vi "Equal Type Comparison.vi"(8 "error in (no error)":errorcluster, 9 "Y":variant, 10 "X":variant) -> (0 "error out":errorcluster, 2 "Equal Types?":bool)   [LabVIEW 2013, in "Caraya.lvlib" / "Assert.lvclass"]
uses:
  classes/Assert/Assert.lvclass
  <vilib>/Utility/VariantDataType/Type.ctl
  <vilib>/Utility/VariantDataType/VariantType.lvlib
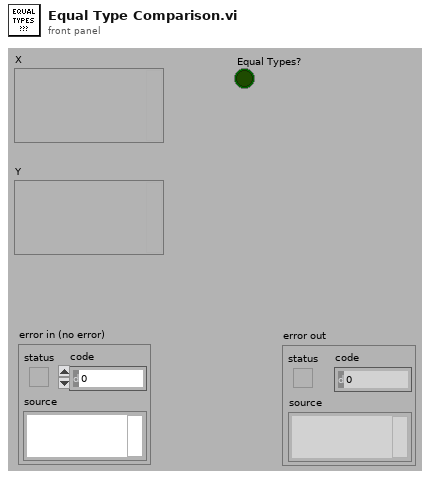
[diagram p1: front panel]
types:
  T1 = typedef "VariantType.lvlib/Type.ctl" = enum8{"Invalid Type", "Void", "I8", "I16", "I32", "I64", "U8", "U16", "U32", "U64", "Single Float", "Double Float", "Extended Float", "Single Complex", "Double Complex", "Extended Complex", "Enum U8", "Enum U16", "Enum U32", "Enum U64", "Single Float With Unit", "Double Float With Unit", "Extended Float With Unit", "Single Complex with Unit", "Double Complex with Unit", "Extended Complex with Unit", "Boolean", "String", "Path", "Picture", "Tag", "Array", "Cluster", "Variant", "LV Variant", "Waveform", "Timestamp", "Digital Waveform", "Digital Data", "ExpressData", "Refnum", "External Data", "VI", "Poly VI", "LabVIEW Class Instance", "Fixed Point"}
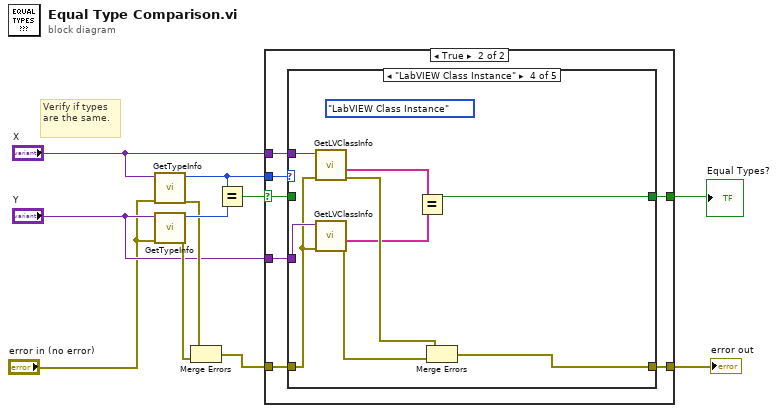
[diagram p0: block diagram]
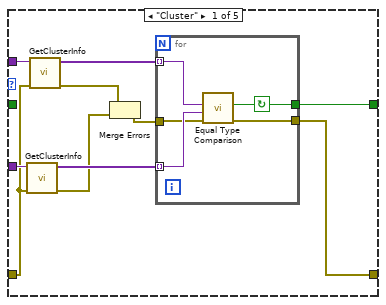
[diagram p3: hidden frame]
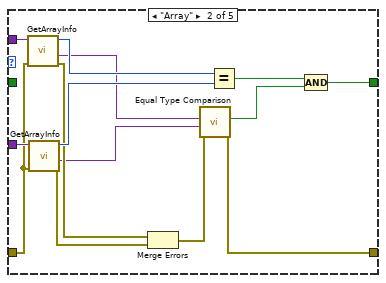
[diagram p4: hidden frame]
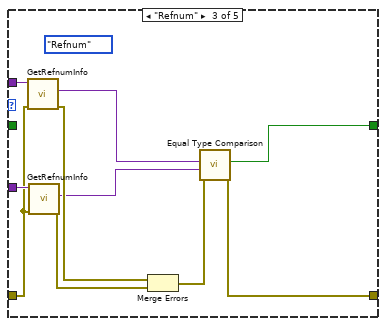
[diagram p5: hidden frame]
diagram:
  # "Verify if types are the same."
  n1 = call <vilib>:"GetTypeInfo.vi"("error in (no error)"="error in (no error)", "Variant"="X") -> ("error out"=w10:errorcluster, "Type Enum"=w7:T1)  [unwired: 5 in, 3 out]
  n2 = call <vilib>:"GetTypeInfo.vi"("error in (no error)"="error in (no error)", "Variant"="Y") -> ("error out"=w9:errorcluster, "Type Enum"=w11:T1)  [unwired: 5 in, 3 out]
  n3 = Merge Errors(w10, w9) -> (w6:errorcluster)
  n4 = Equal?(x=w7, y=w11) -> (x = y?=w8:bool)
  n5 = case shown="True" w8 {
    selector: w8 -> [w13 w19]
    tunnel: [w13 w18] -> w1
    tunnel: w7 -> [_ w20]
    tunnel: "X" -> [_ w17]
    tunnel: "Y" -> [_ w16]
    tunnel: w6 -> [w12 w15]
    tunnel: [w12 w14] -> w2
    frame False {
      # "Not Equal Type"
    }
    frame True {
      n6 = case shown="\"LabVIEW Class Instance\"" w20 {
        tunnel: [w30 w43 w54 w60 w70] -> w18
        tunnel: w19 -> [_ _ _ _ w70]
        tunnel: w17 -> [w29 w49 w57 w68 _]
        tunnel: w16 -> [w27 w48 w53 w67 _]
        tunnel: w15 -> [w25 w44 w51 w66 w69]
        tunnel: [w24 w36 w58 w63 w69] -> w14
        frame "Cluster" {
          n7 = call <vilib>:"GetClusterInfo.vi"("error in (no error)"=w25, "Variant"=w27) -> ("error out"=w21:errorcluster, "Cluster Elements"=w26:variant[])  [unwired: 8 in]
          n8 = call <vilib>:"GetClusterInfo.vi"("error in (no error)"=w25, "Variant"=w29) -> ("error out"=w22:errorcluster, "Cluster Elements"=w28:variant[])  [unwired: 8 in]
          n9 = Merge Errors(w22, w21) -> (w23:errorcluster)
          n10 = for {
            tunnel: [w33] -> w30
            tunnel: w28 -> [w35] mode=indexing
            tunnel: w26 -> [w34] mode=indexing
            tunnel: w23 -> [w32]
            tunnel: [w31] -> w24
            stop <- w33 continue-if-true
            n11 = call "Equal Type Comparison.vi"("error in (no error)"=w32, "Y"=w34, "X"=w35) -> ("error out"=w31:errorcluster, "Equal Types?"=w33:bool)  [unwired: 7 in]
          }
        }
        frame "Array" {
          n12 = call <vilib>:"GetArrayInfo.vi"("error in (no error)"=w44, "Variant"=w49) -> ("error out"=w42:errorcluster, "ArrayElement"=w40:variant, "NDims"=w47:i32)  [unwired: 6 in, 1 out]
          n13 = call <vilib>:"GetArrayInfo.vi"("error in (no error)"=w44, "Variant"=w48) -> ("error out"=w41:errorcluster, "ArrayElement"=w39:variant, "NDims"=w46:i32)  [unwired: 6 in, 1 out]
          n14 = Merge Errors(w42, w41) -> (w37:errorcluster)
          n15 = call "Equal Type Comparison.vi"("error in (no error)"=w37, "Y"=w39, "X"=w40) -> ("error out"=w36:errorcluster, "Equal Types?"=w38:bool)  [unwired: 7 in]
          n16 = Equal?(x=w47, y=w46) -> (x = y?=w45:bool)
          n17 = Compound Arithmetic op=AND(w45, w38) -> (w43:bool)
        }
        frame "Refnum" {
          (unwired) Type."Refnum" ("Type Enum")
          n18 = call <vilib>:"GetRefnumInfo.vi"("error in (no error)"=w51, "Variant"=w57) -> ("error out"=w56:errorcluster, "StrictType"=w55:variant)  [unwired: 6 in, 2 out]
          n19 = call <vilib>:"GetRefnumInfo.vi"("error in (no error)"=w51, "Variant"=w53) -> ("error out"=w52:errorcluster, "StrictType"=w50:variant)  [unwired: 6 in, 2 out]
          n20 = Merge Errors(w56, w52) -> (w59:errorcluster)
          n21 = call "Equal Type Comparison.vi"("error in (no error)"=w59, "Y"=w50, "X"=w55) -> ("error out"=w58:errorcluster, "Equal Types?"=w54:bool)  [unwired: 7 in]
        }
        frame "LabVIEW Class Instance" {
          (unwired) Type."LabVIEW Class Instance" ("Type Enum")
          n22 = call <vilib>:"GetLVClassInfo.vi"("error in (no error)"=w66, "Variant"=w68) -> ("error out"=w65:errorcluster, "Fully Qualified LV Class Name"=w61:string[])  [unwired: 7 in, 1 out]
          n23 = call <vilib>:"GetLVClassInfo.vi"("error in (no error)"=w66, "Variant"=w67) -> ("error out"=w64:errorcluster, "Fully Qualified LV Class Name"=w62:string[])  [unwired: 7 in, 1 out]
          n24 = Equal?(x=w61, y=w62) -> (x = y?=w60:bool)
          n25 = Merge Errors(w65, w64) -> (w63:errorcluster)
        }
        frame Default {
        }
      }
    }
  }
  "Equal Types?" <- w1
  "error out" <- w2
